vi "Set Gain Setting.vi"(0 "RedPitaya connection in":refnum<k5>, 3 "Gain Voltage":enum16{"Low voltage", "High voltage"}(ring), 5 "error in":errorcluster, 8 "Channel #":u16(ring)=1 items=["Channel 1"=1, "Channel 2"=2], 12 "timeout ms (2000)":i32=2000) -> (14 "RedPitaya connection out":refnum<k5>, 19 "error out":errorcluster)   [LabVIEW 2010, in "RedPitaya.lvlib"]
doc: "Set gain settings to HIGH or LOW. This gain is referring to jumper settings on Red Pitaya fast analog inputs."
uses:
  RedPitaya.lvlib
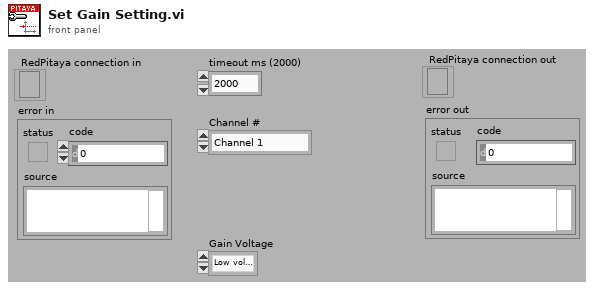
[diagram p1: front panel]
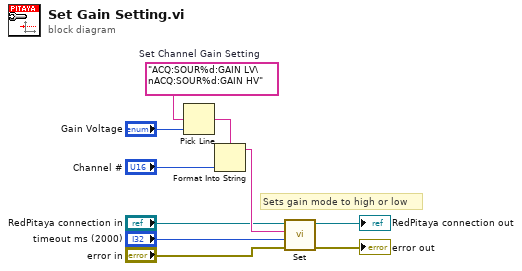
[diagram p0: block diagram]
diagram:
  w3 = "ACQ:SOUR%d:GAIN LV\nACQ:SOUR%d:GAIN HV"  # Set Channel Gain Setting
  # "Sets gain mode to high or low"
  n1 = Pick Line(multi-line string=w3, line index="Gain Voltage") -> (output string=w2:string)  [unwired: 1 in]
  n2 = Format Into String(format string=w2, "Channel #") -> (resulting string=w10:string)  [unwired: 2 in, 1 out]
  n3 = call "Set.vi"("error in"="error in", "timeout ms (2000)"="timeout ms (2000)", "SCPI Message"=w10, "RedPitaya connection in"="RedPitaya connection in") -> ("error out"=→"error out":errorcluster, "RedPitaya connection out"=→"RedPitaya connection out":refnum<k5>)  [unwired: 5 in, 1 out]
